vi "Prepare Update Row Command.vi"(8 "Error In (no error)":errorcluster, 10 "Record":variant) -> (0 "Error Out":errorcluster, 2 "Insert SQL Command":string)   [LabVIEW 2023, in "SQLite DB Operator.lvclass"]
uses:
  SQLite DB Operator.lvclass
  SQLite DB Operator.lvclass/SQLite DB Operator.ctl
  <vilib>/Utility/Data Type/NI_Data Type.lvlib
  <userlib>/_OpenG.lib/array/array.llb/Search 1D Array (String)__ogtk.vi
  <userlib>/_OpenG.lib/array/array.llb/Delete Elements from 1D Array (String)__ogtk.vi
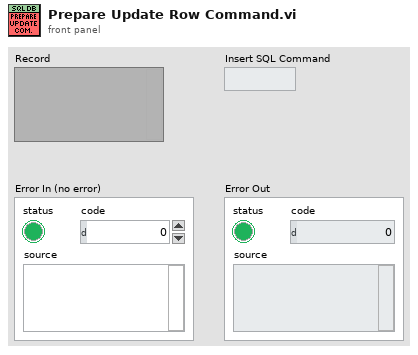
[diagram p1: front panel]
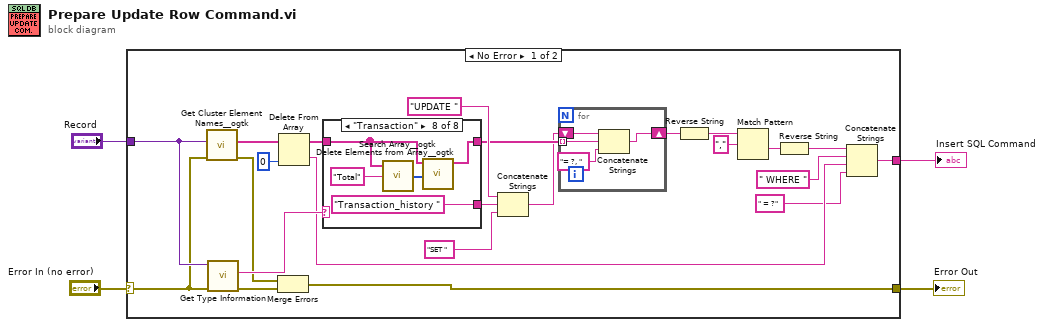
[diagram p0: block diagram]
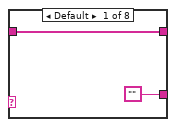
[diagram p2: hidden frame]
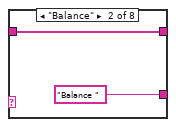
[diagram p3: hidden frame]
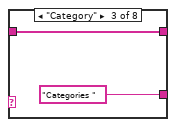
[diagram p4: hidden frame]
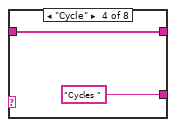
[diagram p5: hidden frame]
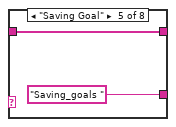
[diagram p6: hidden frame]
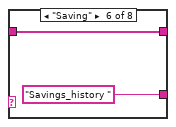
[diagram p7: hidden frame]
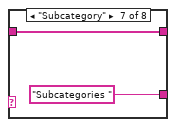
[diagram p8: hidden frame]
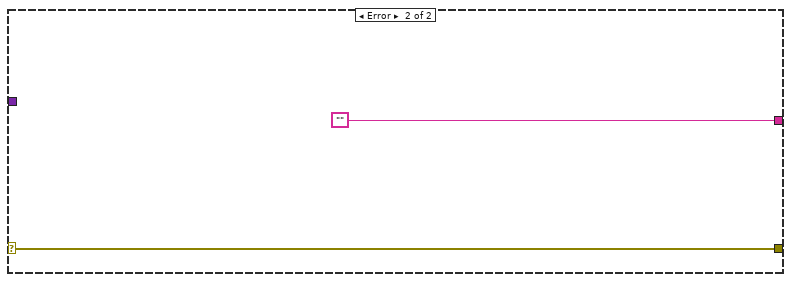
[diagram p9: hidden frame]
diagram:
  n1 = case shown="No Error" "Error In (no error)" {
    selector: "Error In (no error)" -> [w19 w52]
    tunnel: [w25 w52] -> w4
    tunnel: [w5 ""] -> w3
    tunnel: "Record" -> [w20 _]
    frame No Error {
      n2 = call <userlib>:"Get Cluster Element Names__ogtk.vi"("error in (no error)"=w19, "Cluster"=w20) -> ("error out"=w22:errorcluster, "Element Names"=w21:string[])  [unwired: 8 in]
      n3 = call <vilib>:"Get Type Information.vi"("error in (no error)"=w19, "variant"=w20) -> ("error out"=w23:errorcluster, "name"=w27:string)  [unwired: 5 in, 3 out]
      n4 = Merge Errors(w22, w23) -> (w25:errorcluster)
      n5 = Delete From Array(array=w21, index=0) -> (deleted portion=w7:string, array with subset deleted=w16:string[])  [unwired: 1 in]
      n6 = case shown="\"Transaction\"" w27 {
        tunnel: ["" "Balance " ("string") "Categories " ("string") "Cycles " ("string") "Saving_goals " ("string") "Savings_history " ("string") "Subcategories " ("string") "Transaction_history " ("string")] -> w24
        tunnel: w16 -> [w32 w34 w36 w38 w40 w42 w44 w47]
        tunnel: [w32 w34 w36 w38 w40 w42 w44 w46] -> w17
        frame Default {
        }
        frame "Balance" {
        }
        frame "Category" {
        }
        frame "Cycle" {
        }
        frame "Saving Goal" {
        }
        frame "Saving" {
        }
        frame "Subcategory" {
        }
        frame "Transaction" {
          n7 = call-poly <userlib>:"Search Array__ogtk.vi"("Array"=w47, "Element Data"="Total") -> ("Indices of Elements"=w48:i32[])  [unwired: 7 in]
          n8 = call-poly <userlib>:"Delete Elements from Array__ogtk.vi"("indices"=w48, "array"=w47) -> ("array w/ subset deleted"=w46:string[])  [unwired: 8 in, 1 out]
        }
      }
      n9 = Concatenate Strings("UPDATE ", w24, "SET ") -> (w10:string)
      n10 = for {
        tunnel: w17 -> [w30] mode=indexing
        shift-right: [w29] -> w14
        shift-left: w10 -> [w31]
        n11 = Concatenate Strings(w31, w30, "= ?, " ("string")) -> (w29:string)
      }
      n12 = Reverse String(1:w14) -> (0:w13:string)
      n13 = Match Pattern(string=w13, regular expression=",") -> (after substring=w11:string)  [unwired: 1 in, 3 out]
      n14 = Reverse String(1:w11) -> (0:w9:string)
      n15 = Concatenate Strings(w9, " WHERE ", w7, " = ?" ("string")) -> (w5:string)
    }
    frame Error {
    }
  }
  "Error Out" <- w4
  "Insert SQL Command" <- w3
